vi "4-20mA Module (Main).vi"(7 "Name of Parent Panel":string="Main.vi", 9 "New Center Coords":T1={"Horizontal"=470, "Vertical"=200}, 10 "Config":variant, 11 "Main UI Message Queue":refnum<queue>) -> ()   [LabVIEW 2018, in "4-20mA Module.lvlib"]
doc: "This Continuous Measurement sample project is based on the Queued Message Handler template.\n\nThe Event Handling Loop generates messages based on user interface actions.\n\nThe Message Handling Loop processes messages generated by the Event Handling Loop, or by other messages. There are also Acquisition and Logging message handling loop subVIs, and a chart updating loop."
uses:
  4-20mA Module.lvlib
  support/Message Queue/Message Cluster.ctl
  <vilib>/Utility/miscctls.llb/LVPoint32TypeDef.ctl
  controls/UI Data.ctl
  controls/UI State.ctl
  Controls/4-20mA Module State Cluster.ctl
  Controls/4-20mA Module Config Cluster.ctl
  Controls/4-20mA Module Settings Cluster.ctl
  Pressure Transmitter/Pressure Transmitter Device Settings.ctl
  Pressure Reg Module/Pressure Regulator Device Settings.ctl
  Measure Instrument/State Enum.ctl
  Controls/4-20mA Display Cluster.ctl
  Tag VIs/Tag FGV Operation Enum.ctl
  Sequencing/Squence Update Cluster.ctl
  support/Message Queue/Enqueue Message (Single).vi
  <vilib>/Utility/error.llb/Error Cluster From Error Code.vi
  <vilib>/ErrorRing/Error Ring.xnode
  support/User Event - Stop/User Event - Stop.lvlib
  support/Support Library.lvlib
  support/Message Queue/Message Queue.lvlib
  Measure Instrument/4-20mA Module Engine.lvlib
  Sequencing/Sequencing Library.lvlib
  Pressure Transmitter/Pressure Transmitter Library.lvlib
  Pressure Reg Module/Pressure Regulator Library.lvlib
  Shared Variables/Dynamic Shared Variables.lvlib
  Measure Instrument/Feed Module Engine.lvlib
  support/Command Log VIs/Command Logging.lvlib
panel:
  in  "Settings Dialog Button":bool
  out "Image Status":u16(ring)=2
  out "Input Channel":string
  out "Output":dbl caption="mA" format="%.2f"
  out "Input":dbl caption="mA" format="%.2f"
  out "Log File path":path
  out "Status":string
  in  "Exit":bool
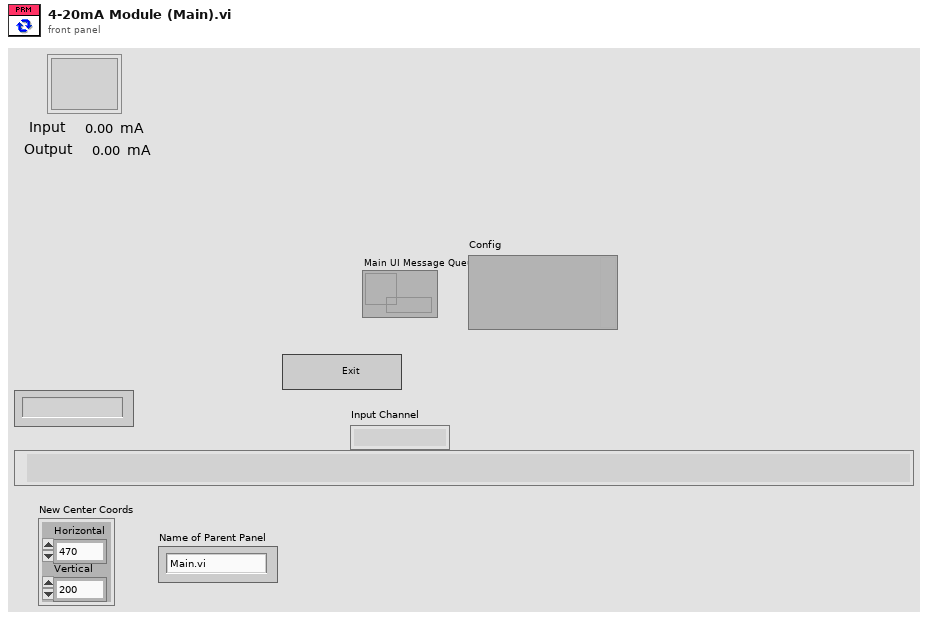
[diagram p1: front panel]
types:
  T1 = typedef "LVPoint32TypeDef.ctl" = cluster{"Horizontal":i32, "Vertical":i32}
  T2 = typedef "4-20mA Module.lvlib/4-20mA Module Config Cluster.ctl" = cluster{"GUID":string, "Drop Coords":T1, "Process Name":string, "Settings":T3, "Settings Load Count":i32}
  T3 = typedef "4-20mA Module.lvlib/4-20mA Module Settings Cluster.ctl" = cluster{"Cycle Period":dbl, "PID 2 Parameters":cluster{"Input Device":enum16{"Default", "4-20mA"}, "Output Device":enum16{"Default", "Equilibar Pressure Reg", "Flow Regulator"}, "Setpoint":dbl, "PID gains":cluster{"proportional gain (Kc)":dbl, "integral time (Ti, min)":dbl, "derivative time (Td, min)":dbl}, "output range":cluster{"output low":dbl, "output high":dbl}}, "Manual Entry":dbl, "Auto?":bool, "4-20mA Input Settings":T4, "4-20mA Out Settings":T5, "Input Channel Tag Name ":string}
  T4 = typedef "Pressure Transmitter Library.lvlib/Pressure Transmitter Device Settings.ctl" = cluster{"Input Channel ":u16}
  T5 = typedef "Pressure Regulator Library.lvlib/Pressure Regulator Device Settings.ctl" = cluster{"Output DAQ Task":refnum<k21>}
  T6 = typedef "4-20mA Module.lvlib/4-20mA Module State Cluster.ctl" = cluster{"PRM Config":T2, "State":T7, "Start Time":timestamp, "Current Time":timestamp, "First Iteration":bool, "Data":cluster{"4-20mA Input":dbl, "PID 2 Process Variable":dbl, "PID 2 Output":dbl, "4-20mA Output":dbl}}
  T7 = typedef "Feed Module.lvlib/Feed Module Engine.lvlib/State Enum.ctl" = enum16{"Measuring", "Idle", "Paused"}
  T8 = typedef "UI State.ctl" = enum16{"Idle", "Acquiring and Logging", "Waiting for Exit", "Waiting for Exit (Acq Stopped)", "Waiting for Exit (Log Stopped)", "Waiting for Stop", "Waiting for Stop (Acq Stopped)", "Waiting for Stop (Log Stopped)"}
  T9 = typedef "UI Data.ctl" = cluster{"Start Ref":refnum<vi>, "Trigger Ref":refnum<vi>, "Stop Ref":refnum<vi>, "Settings Ref":refnum<vi>, "Status Ref":refnum<vi>, "Exit Ref":refnum<vi>, "Data Ref":refnum<vi>}
  T10 = typedef "4-20mA Module.lvlib/4-20mA Message Queues.ctl" = cluster{"UI":refnum<queue>, "Engine":refnum<queue>, "PR Display":refnum<queue>, "Setting Display":refnum<queue>}
  T11 = typedef "4-20mA Module.lvlib/4-20mA Display Cluster.ctl" = cluster{"Input 4-20":dbl, "Output 4-20":dbl, "Cycle Period":dbl, "Status":enum16{"Off", "On", "Not Initialized"}}
  T12 = typedef "Tag FGV Operation Enum.ctl" = enum16{"Init", "Set Notification Queue", "Create Tag", "Commit", "Write Tag (Numeric)", "Write Tag (Boolean)", "Read All Tags", "Read One Tag", "Delete Tag Category", "Set Alarm Parameters (Numeric)", "Set Alarm Parameters (Boolean)", "Enable All Alarms", "Disable All Alarms", "Delete All Tags", "Read Alarms", "Ack Alarm"}
  T13 = cluster{"Shift":bool, "Ctrl":bool, "Alt":bool, "Cmd":bool, "Opt":bool}
  T14 = typedef "Sequencing Library.lvlib/Squence Update Cluster.ctl" = cluster{"Auto?":bool, "Manual Entry":dbl, "Setpoint":dbl}
  T15 = enum8{"Enabled", "Disabled", "Disabled and Grayed Out"}
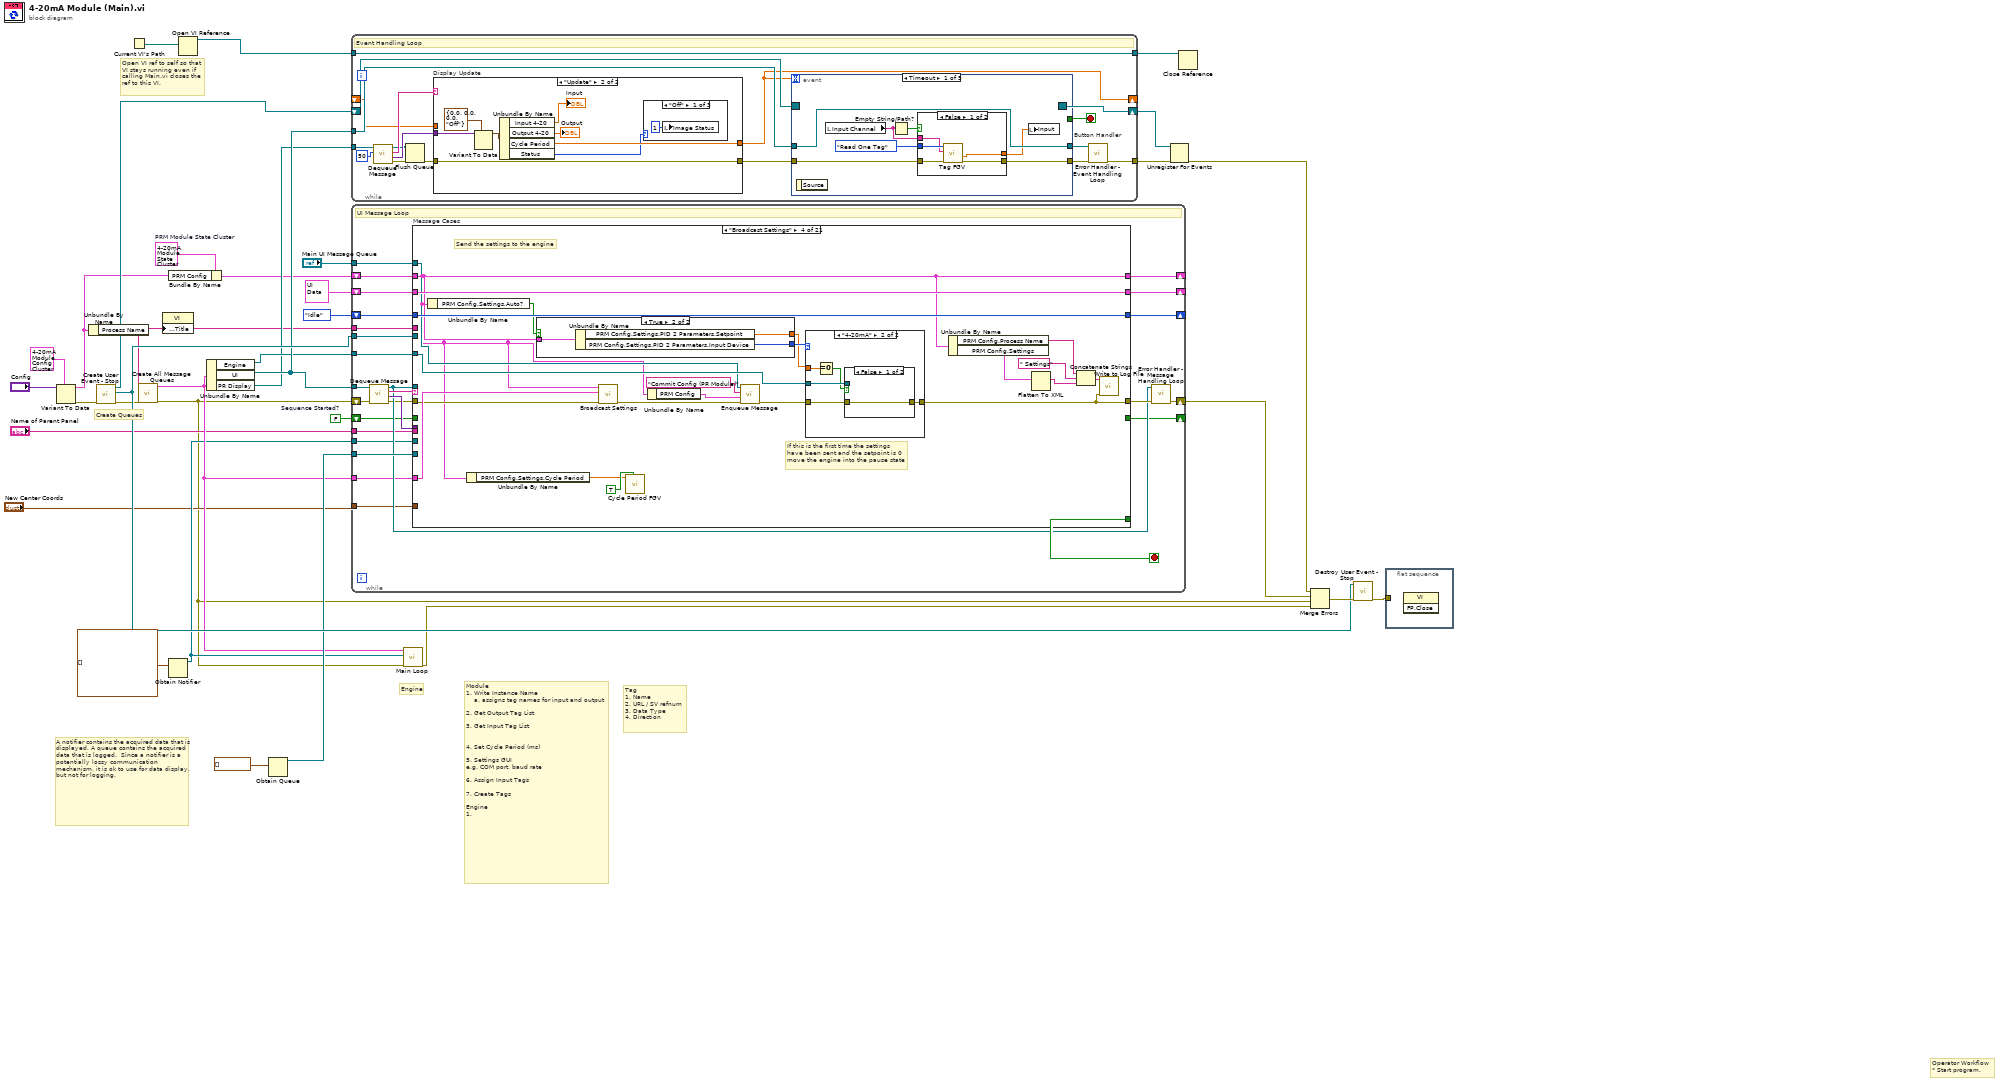
[diagram p0: block diagram]
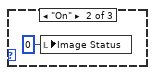
[diagram p3: hidden frame]
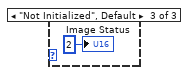
[diagram p4: hidden frame]
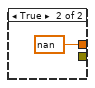
[diagram p5: hidden frame]
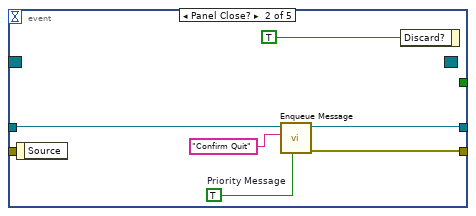
[diagram p6: hidden frame]
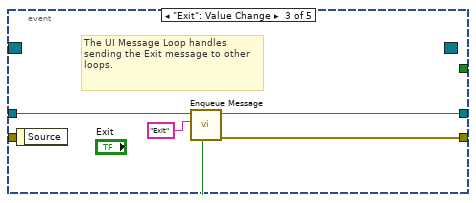
[diagram p7: hidden frame]
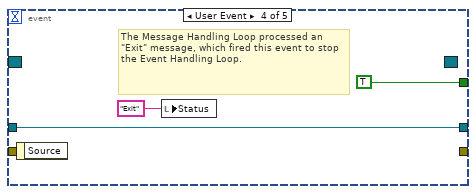
[diagram p8: hidden frame]
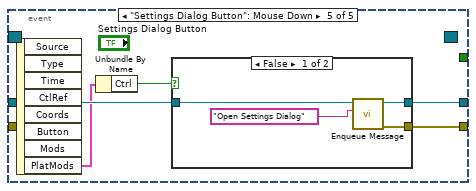
[diagram p9: hidden frame]
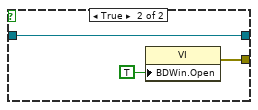
[diagram p10: hidden frame]
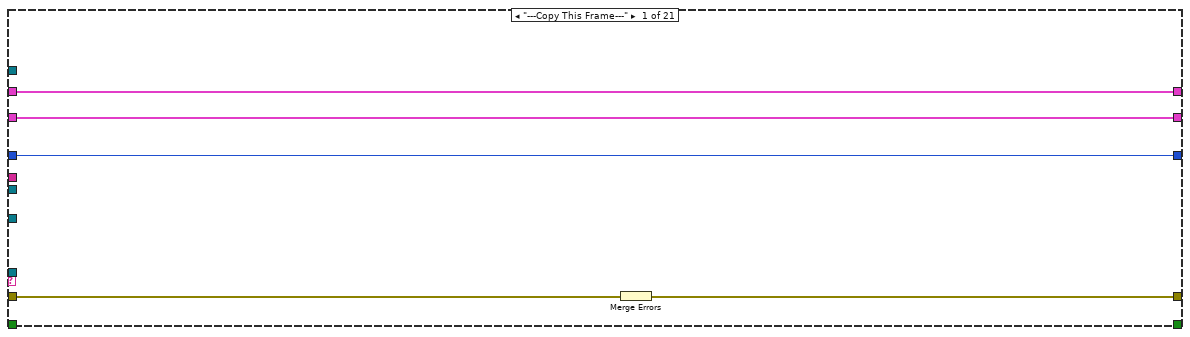
[diagram p11: hidden frame]
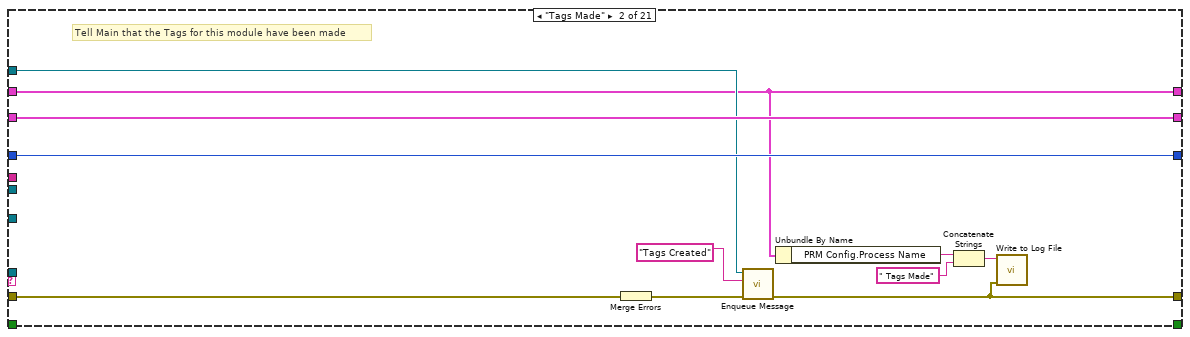
[diagram p12: hidden frame]
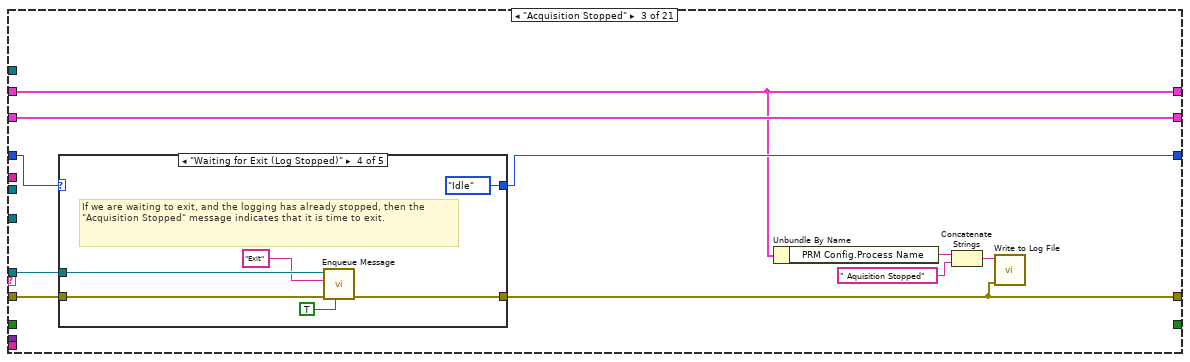
[diagram p13: hidden frame]
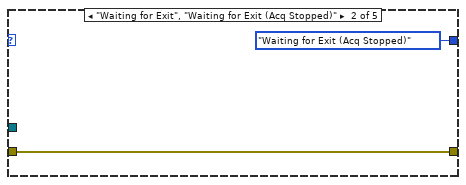
[diagram p15: hidden frame]
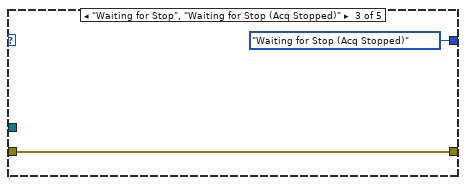
[diagram p16: hidden frame]
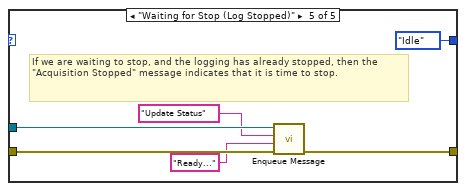
[diagram p17: hidden frame]
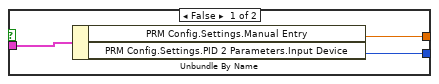
[diagram p18: hidden frame]
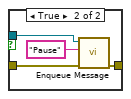
[diagram p20: hidden frame]
diagram:
  w5 = FALSE  # Sequence Started?
  w11 = T6 {"PRM Config"={"GUID"="", "Drop Coords"={"Horizontal"=0, "Vertical"=0}, "Process Name"="", "Settings"={"Cycle Period"=500.0, "PID 2 Parameters"={"Input Device"=enum."Default", "Output Device"=enum."Default", "Setpoint"=0.0, "PID gains"={"proportional gain (Kc)"=1.0, "integral time (Ti, min)"=0.01, "derivative time (Td, min)"=0.0}, "output range"={"output low"=0.0, "output high"=100.0}}, "Manual Entry"=0.0, "Auto?"=TRUE, "4-20mA Input Settings"={"Input Channel "=0}, "4-20mA Out Settings"={"Output DAQ Task"=""}, "Input Channel Tag Name "=""}, "Settings Load Count"=0}, "State"=enum."Idle", "Start Time"=timestamp(0 s since 1904-01-01), "Current Time"=timestamp(0 s since 1904-01-01), "First Iteration"=FALSE, "Data"={"4-20mA Input"=0.0, "PID 2 Process Variable"=0.0, "PID 2 Output"=0.0, "4-20mA Output"=0.0}}  # PRM Module State Cluster
  # "Create Queues"
  # "Open VI ref to self so that\nVI stays running even if\ncalling Main.vi closes the\nref to this VI."
  # "Engine"
  # "Operator Workflow\n* Start program."
  # "Module \n1. Write Instance Name\n    a. assigns tag names for input and output\n\n2. Get Output Tag List\n\n3. Get Input Tag List\n\n\n4. Set Cycle Period (ms)\n\n5. Settings GUI\ne.g. COM port, baud rate\n\n6. Assign Input Tags\n\n7. Create Tags\n\nEngine\n1."
  # "Tag\n1. Name\n2. URL / SV refnum\n3. Data Type\n4. Direction"
  # "A notifier contains the acquired data that is displayed. A queue contains the acquired data that is logged.  Since a notifier is a potentially lossy communication mechanism, it is ok to use for data display, but not for logging."
  n1 = Variant To Data(type=T2 {"GUID"="", "Drop Coords"={"Horizontal"=0, "Vertical"=0}, "Process Name"="", "Settings"={"Cycle Period"=500.0, "PID 2 Parameters"={"Input Device"=enum."Default", "Output Device"=enum."Default", "Setpoint"=0.0, "PID gains"={"proportional gain (Kc)"=1.0, "integral time (Ti, min)"=0.01, "derivative time (Td, min)"=0.0}, "output range"={"output low"=0.0, "output high"=100.0}}, "Manual Entry"=0.0, "Auto?"=TRUE, "4-20mA Input Settings"={"Input Channel "=0}, "4-20mA Out Settings"={"Output DAQ Task"=""}, "Input Channel Tag Name "=""}, "Settings Load Count"=0} ("Feed Module Config"), Variant="Config") -> (data=w13:T2, error out=w14:errorcluster)  [unwired: 1 in]
  n2 = Unbundle By Name(w13) -> ("Process Name"=w8:string)
  n3 = call "Create User Event - Stop.vi"("error in (no error)"=w14) -> ("error out"=w30:errorcluster, "User Event - Stop"=w31:refnum<user-event>, "Stop Event Registration Refnum"=w32:refnum<event-registration>)  [unwired: 8 in]
  n4 = Current VI's Path() -> (path=w15:path)
  n5 = call "Create All Message Queues.vi"("error in (no error)"=w30, "Process Name"=w8) -> ("error out"=w4:errorcluster, "Message Queues"=w19:T10)  [unwired: 8 in]
  n6 = property class="VI"("Front Panel.Title"=w8) -> ()  [unwired: 2 in, 2 out]
  n7 = Bundle By Name(cluster=w11, "PRM Config"=w13) -> (w1:T6)
  n8 = Obtain Notifier(notification data type=waveform(dbl)[] []) -> (notifier out=w18:refnum<notifier>)  [unwired: 3 in, 2 out]
  n9 = Open VI Reference(vi path=w15) -> (vi reference=w16:refnum<vi>)  [unwired: 5 in, 1 out]
  n10 = Unbundle By Name(w19) -> ("Engine"=w22:refnum<queue>, "UI"=w26:refnum<queue>, "PR Display"=w10:refnum<queue>)
  n11 = Obtain Queue(element data type=waveform(dbl)[] []) -> (queue out=w21:refnum<queue>)  [unwired: 4 in, 2 out]
  n12 = while {
    tunnel: w26 -> [w47]
    tunnel: [w49] -> w34
    shift-right: [w48] -> w28
    shift-left: w32 -> [w53]
    tunnel: [w46] -> w17
    tunnel: w16 -> [w46]
    tunnel: w10 -> [w45]
    shift-right: [w42] -> _
    shift-left: _ -> [w41]
    stop <- w52 stop-if-true
    # "Event Handling Loop"
    n13 = call "Dequeue Message.vi"("timeout in ms (-1)"=50, "Message Queue"=w45) -> ("error out"=w38:errorcluster, "Message Data"=w43:variant, "Message"=w44:string, "dup Message Queue"=w39:refnum<queue>)  [unwired: 6 in]
    n14 = Flush Queue(queue=w39, error in (no error)=w38) -> (error out=w36:errorcluster)  [unwired: 2 out]
    n15 = case "Display Update" shown="\"Update\"" w44 {
      tunnel: w43 -> [_ w63]
      tunnel: [w55 w59] -> w42
      tunnel: w41 -> [w55 _]
      tunnel: [w54 w57] -> w37
      tunnel: w36 -> [w54 w57]
      frame "False", Default {
      }
      frame "Update" {
        n16 = Variant To Data(type=T11 {"Input 4-20"=0.0, "Output 4-20"=0.0, "Cycle Period"=0.0, "Status"=enum."Off"} ("PRM Display Cluster"), Variant=w63) -> (data=w62:T11)  [unwired: 1 in, 1 out]
        n17 = Unbundle By Name(w62) -> ("Input 4-20"=→"Input":dbl, "Output 4-20"=→"Output":dbl, "Cycle Period"=w59:dbl, "Status"=w56:enum16{"Off", "On", "Not Initialized"})
        n18 = case shown="\"Off\"" w56 {
          frame "Off" {
            n19 = local write "Image Status"(u16 1 ("Ring")) -> ()
          }
          frame "On" {
            n20 = local write "Image Status"(u16 0 ("Ring")) -> ()
          }
          frame "Not Initialized", Default {
            "Image Status" <- u16 2 ("Ring")
          }
        }
      }
    }
    n21 = event "Button Handler" shown="[0] Timeout" {
      selector: w53 -> [_ _ _ _ _]
      dyn-events: [_ _ _ _ _] -> w48
      timeout: w42 -> [_ _ _ _ _]
      tunnel: [_ _ _ TRUE ("Discard?") _] -> w52
      tunnel: w47 -> [w73 w82 w87 w91 w96]
      tunnel: [w67 w80 w90 _ w98] -> w50
      tunnel: [w73 w81 w86 w91 w97] -> w51
      tunnel: w37 -> [w68 _ _ _ _]
      event Timeout {
        n22 = event-data() -> ()  [unwired: 1 in, 1 out]
        n23 = local read "Input Channel"() -> (w69:string)
        n24 = Empty String/Path?(string/path=w69) -> (empty?=w72:bool)
        n25 = case shown="False" w72 {
          tunnel: Tag_FGV_Operation_Enum."Read One Tag" ("Operation") -> [w78 _]
          tunnel: [w77 nan ("Tag Value")] -> w70
          tunnel: [w76 _] -> w67
          tunnel: w69 -> [w75 _]
          tunnel: w68 -> [w74 _]
          frame False {
            n26 = call "Tag FGV.vi"("error in (no error)"=w74, "Tag Name"=w75, "Operation"=w78) -> ("error out"=w76:errorcluster, "Tag Value"=w77:dbl)  [unwired: 3 in, 4 out]
          }
          frame True {
          }
        }
        n27 = local write "Input"(w70) -> ()
      }
      event Panel Close? {
        w83 = TRUE  # Priority Message
        n28 = event-data() -> ()  [unwired: 1 in, 1 out]
        n29 = call-poly "Enqueue Message.vi"("Priority Message? (F)"=w83, "Message"="Confirm Quit", "Message Queue"=w82) -> ("error out"=w80:errorcluster, "dup Message Queue"=w81:refnum<queue>)  [unwired: 7 in]
        n30 = event-data("Discard?"=TRUE) -> ()  [unwired: 1 in, 1 out]
      }
      event "Exit": Value Change {
        w88 = TRUE  # Priority Message
        # "The UI Message Loop handles sending the Exit message to other loops."
        n31 = event-data() -> ()  [unwired: 1 in, 1 out]
        n32 = call-poly "Enqueue Message.vi"("Priority Message? (F)"=w88, "Message"="Exit", "Message Queue"=w87) -> ("error out"=w90:errorcluster, "dup Message Queue"=w86:refnum<queue>)  [unwired: 7 in]
      }
      event User Event {
        # "The Message Handling Loop processed an \"Exit\" message, which fired this event to stop the Event Handling Loop."
        n33 = event-data() -> ()  [unwired: 1 in, 1 out]
        n34 = local write "Status"("Exit" ("Exit String")) -> ()
      }
      event "Settings Dialog Button": Mouse Down {
        n35 = event-data() -> ("PlatMods"=w95:T13)  [unwired: 1 in, 7 out]
        n36 = Unbundle By Name(w95) -> ("Ctrl"=w94:bool)
        n37 = case shown="False" w94 {
          tunnel: [w102 w103] -> w98
          tunnel: [w101 w104] -> w97
          tunnel: w96 -> [w100 w104]
          frame False {
            n38 = call-poly "Enqueue Message.vi"("Message"="Open Settings Dialog", "Message Queue"=w100) -> ("error out"=w102:errorcluster, "dup Message Queue"=w101:refnum<queue>)  [unwired: 8 in]
          }
          frame True {
            n39 = property class="VI"("BDWin.Open"=TRUE ("Block Diagram Window:Open")) -> (error out=w103:errorcluster)  [unwired: 2 in, 1 out]
          }
        }
      }
    }
    n40 = call "Error Handler - Event Handling Loop.vi"("error in (no error)"=w50, "Message Queue"=w51) -> ("dup error in"=w49:errorcluster)  [unwired: 8 in, 1 out]
  }
  n41 = while {
    tunnel: w26 -> [w126]
    tunnel: w31 -> [w130]
    shift-right: [w121] -> w35
    shift-left: w4 -> [w129]
    shift-right: [w124] -> _
    shift-left: T9 {"Start Ref"=refnum, "Trigger Ref"=refnum, "Stop Ref"=refnum, "Settings Ref"=refnum, "Status Ref"=refnum, "Exit Ref"=refnum, "Data Ref"=refnum} ("Measurement UI Controls") -> [w125]
    tunnel: w18 -> [w111]
    tunnel: w21 -> [w123]
    shift-right: [w119] -> _
    shift-left: UI_State."Idle" ("UI State") -> [w113]
    tunnel: w22 -> [w118]
    tunnel: w19 -> [w110]
    tunnel: "Main UI Message Queue" -> [w114]
    tunnel: "Name of Parent Panel" -> [w117]
    tunnel: w8 -> [w116]
    tunnel: "New Center Coords" -> [w115]
    shift-right: [w108] -> _
    shift-left: w5 -> [w109]
    shift-right: [w106] -> _
    shift-left: w1 -> [w107]
    stop <- w131 stop-if-true
    # "UI Message Loop"
    n42 = call "Dequeue Message.vi"("error in (no error)"=w129, "Message Queue"=w126) -> ("error out"=w112:errorcluster, "Message Data"=w127:variant, "Message"=w128:string, "dup Message Queue"=w120:refnum<queue>)  [unwired: 6 in]
    n43 = case "Message Cases" shown="\"Broadcast Settings\"" w128 {
      selector: w128 -> [_ _ _ _ _ _ _ _ _ _ _ _ _ _ _ _ _ _ _ _ w565]
      tunnel: w120 -> [_ _ w153 _ w222 _ w278 w294 w326 w350 _ w388 w409 w419 w452 w472 _ _ w542 _ _]
      tunnel: w112 -> [w136 w147 w154 w192 w221 w248 w263 w293 w329 w354 w373 w383 _ w420 w449 w470 w496 w510 w527 w556 _]
      tunnel: [w135 w138 w149 w179 w216 w249 w255 w282 w317 w332 w373 w375 w396 w415 w451 w463 w502 w516 w543 w557 w566] -> w122
      tunnel: [_ _ _ _ _ _ _ _ _ TRUE _ _ _ _ _ _ _ _ _ _ _] -> w131
      tunnel: w127 -> [_ _ _ _ _ w251 _ _ w328 w338 _ _ w407 _ _ _ _ _ _ w555 _]
      tunnel: w130 -> [_ _ _ _ _ _ _ _ _ w353 _ _ _ _ _ _ _ _ _ _ _]
      tunnel: w125 -> [w134 w146 w157 w197 w224 w253 w275 w291 w330 w351 w372 w384 w413 w423 w457 w486 w501 w515 w539 w552 w567]
      tunnel: [w134 w146 w157 w197 w224 w253 w275 w291 w330 w351 w371 w384 w413 w423 w457 w486 w501 w515 w539 w552 w567] -> w124
      tunnel: w123 -> [_ _ _ _ _ _ _ _ _ w345 _ _ _ _ _ _ _ _ _ _ _]
      tunnel: w113 -> [w133 w145 w156 w196 w223 w247 w264 _ w321 _ _ _ w412 w422 w442 _ _ _ w528 w547 w564]
      tunnel: [w133 w145 w155 w196 w220 w247 w265 UI_State."Acquiring and Logging" ("UI State") w321 UI_State."Idle" ("UI State") UI_State."Idle" ("UI State") UI_State."Idle" ("UI State") w412 w421 w442 UI_State."Acquiring and Logging" ("UI State") UI_State."Acquiring and Logging" ("UI State") UI_State."Acquiring and Logging" ("UI State") w529 w547 w564] -> w119
      tunnel: w118 -> [_ _ _ w191 _ _ w262 _ _ w343 _ _ _ _ _ _ w499 w513 w526 _ _]
      tunnel: w117 -> [_ _ _ _ _ _ _ _ _ _ _ w382 _ _ _ _ _ _ _ _ _]
      tunnel: w116 -> [_ _ _ _ _ _ _ _ _ _ _ w379 _ _ _ _ _ _ _ _ _]
      tunnel: w115 -> [_ _ _ _ _ _ _ _ _ _ _ w381 _ _ _ _ _ _ _ _ _]
      tunnel: w114 -> [_ w143 _ w184 _ _ _ _ _ w336 _ _ _ _ _ _ _ _ _ _ _]
      tunnel: w111 -> [_ _ _ _ _ _ _ _ _ w349 _ _ _ _ _ _ _ _ _ _ _]
      tunnel: w110 -> [_ _ _ w195 _ _ _ _ _ _ _ _ _ _ w443 _ _ _ _ _ _]
      tunnel: w107 -> [w132 w137 w148 w178 w215 w246 w254 w281 w316 w331 w364 w374 w411 w414 w450 w464 w494 w508 w522 w546 w563]
      tunnel: w109 -> [_ _ _ _ _ _ _ w290 _ _ _ _ _ _ _ _ _ _ _ _ _]
      tunnel: [_ _ _ _ _ _ _ w287 _ _ _ _ _ _ _ _ _ _ _ _ _] -> w108
      tunnel: [w132 w137 w148 w178 w215 w246 w254 w281 w316 w331 w364 w374 w395 w414 w445 w464 w494 w508 w522 w546 w563] -> w106
      frame "---Copy This Frame---" {
        # "Duplicate this frame when creating new messages.  Change this comment in the duplicated frame to describe this message."
        n44 = Merge Errors(w136) -> (w135:errorcluster)
      }
      frame "Tags Made" {
        # "Tell Main that the Tags for this module have been made"
        # "Duplicate this frame when creating new messages.  Change this comment in the duplicated frame to describe this message."
        n45 = Merge Errors(w147) -> (w142:errorcluster)
        n46 = call-poly "Enqueue Message.vi"("error in (no error)"=w142, "Message"="Tags Created", "Message Queue"=w143) -> ("error out"=w138:errorcluster)  [unwired: 7 in, 1 out]
        n47 = Unbundle By Name(w137) -> ("PRM Config.Process Name"=w141:string)
        n48 = Concatenate Strings(w141, " Tags Made" ("text")) -> (w139:string)
        n49 = call "Write to Log File.vi"("error in"=w138, "text"=w139) -> ()  [unwired: 9 in, 1 out]
      }
      frame "Acquisition Stopped" {
        # "Logic for determining what action to take when the acquisition has stopped."
        n50 = case shown="\"Waiting for Exit (Log Stopped)\"" w156 {
          selector: w156 -> [w159 _ _ _ _]
          tunnel: [w159 UI_State."Waiting for Exit (Acq Stopped)" ("UI State") UI_State."Waiting for Stop (Acq Stopped)" ("UI State") UI_State."Idle" ("UI State") UI_State."Idle" ("UI State")] -> w155
          tunnel: w154 -> [w158 w160 w162 w168 w174]
          tunnel: [w158 w160 w162 w167 w173] -> w149
          tunnel: w153 -> [_ _ _ w166 w172]
          frame Default {
          }
          frame "Waiting for Exit", "Waiting for Exit (Acq Stopped)" {
          }
          frame "Waiting for Stop", "Waiting for Stop (Acq Stopped)" {
          }
          frame "Waiting for Exit (Log Stopped)" {
            # "If we are waiting to exit, and the logging has already stopped, then the \"Acquisition Stopped\" message indicates that it is time to exit."
            n51 = call-poly "Enqueue Message.vi"("Priority Message? (F)"=TRUE, "error in (no error)"=w168, "Message"="Exit", "Message Queue"=w166) -> ("error out"=w167:errorcluster)  [unwired: 6 in, 1 out]
          }
          frame "Waiting for Stop (Log Stopped)" {
            # "If we are waiting to stop, and the logging has already stopped, then the \"Acquisition Stopped\" message indicates that it is time to stop."
            n52 = call-poly "Enqueue Message.vi"("error in (no error)"=w174, "Message Data"="Ready..." ("Message"), "Message"="Update Status", "Message Queue"=w172) -> ("error out"=w173:errorcluster)  [unwired: 6 in, 1 out]
          }
        }
        n53 = Unbundle By Name(w148) -> ("PRM Config.Process Name"=w152:string)
        n54 = Concatenate Strings(w152, " Aquisition Stopped" ("text")) -> (w150:string)
        n55 = call "Write to Log File.vi"("error in"=w149, "text"=w150) -> ()  [unwired: 9 in, 1 out]
      }
      frame "Broadcast Settings" {
        # "If this is the first time the settings\nhave been sent and the setpoint is 0 \nmove the engine into the pause state"
        # "Send the settings to the engine"
        # "Send the 'Update Settings' message to the Logging and Acquisition message loops."
        n56 = Unbundle By Name(w178) -> ("PRM Config.Settings.Auto?"=w188:bool)
        n57 = Unbundle By Name(w178) -> ("PRM Config.Settings.Cycle Period"=w193:dbl)
        n58 = case shown="True" w188 {
          tunnel: [w198 w203] -> w190
          tunnel: [w199 w202] -> w189
          tunnel: w178 -> [w200 w201]
          frame False {
            n59 = Unbundle By Name(w200) -> ("PRM Config.Settings.Manual Entry"=w199:dbl, "PRM Config.Settings.PID 2 Parameters.Input Device"=w198:enum16{"Default", "4-20mA"})
          }
          frame True {
            n60 = Unbundle By Name(w201) -> ("PRM Config.Settings.PID 2 Parameters.Setpoint"=w202:dbl, "PRM Config.Settings.PID 2 Parameters.Input Device"=w203:enum16{"Default", "4-20mA"})
          }
        }
        n61 = call "Broadcast Settings.vi"("error in (no error)"=w192, "Message Queues"=w195, "PRM Module State Cluster"=w178) -> ("error out"=w186:errorcluster)  [unwired: 8 in]
        n62 = call "Cycle Period FGV.vi"("Write"=TRUE, "Cycle Period In (ms)"=w193) -> ()  [unwired: 8 in, 2 out]
        n63 = Unbundle By Name(w178) -> ("PRM Config"=w183:T2)
        n64 = call-poly "Enqueue Message.vi"("error in (no error)"=w186, "Message Data"=w183, "Message"="Commit Config (PR Module)", "Message Queue"=w184) -> ("error out"=w185:errorcluster)  [unwired: 6 in, 1 out]
        n65 = case shown="\"4-20mA\"" w190 {
          tunnel: w185 -> [w204 w209]
          tunnel: w191 -> [_ w208]
          tunnel: [w204 w207] -> w179
          tunnel: w189 -> [_ w206]
          frame "Default", Default {
          }
          frame "4-20mA" {
            n66 = Equal To 0?(x=w206) -> (x = 0?=w205:bool)
            n67 = case shown="False" w205 {
              tunnel: w209 -> [w210 w214]
              tunnel: w208 -> [_ w213]
              tunnel: [w210 w212] -> w207
              frame False {
              }
              frame True {
                n68 = call-poly "Enqueue Message.vi"("error in (no error)"=w214, "Message"="Pause", "Message Queue"=w213) -> ("error out"=w212:errorcluster)  [unwired: 7 in, 1 out]
              }
            }
          }
        }
        n69 = Unbundle By Name(w178) -> ("PRM Config.Process Name"=w182:string, "PRM Config.Settings"=w177:T3)
        n70 = Flatten To XML(anything=w177) -> (xml string=w176:string)
        n71 = Concatenate Strings(w182, " Settings" ("text"), w176) -> (w180:string)
        n72 = call "Write to Log File.vi"("error in"=w179, "text"=w180) -> ()  [unwired: 9 in, 1 out]
      }
      frame "Confirm Quit" {
        # "Confirm Quit - Message that can confirm whether or not the user wants to exit the application."
        n73 = case shown="\"Acquiring and Logging\"" w223 {
          tunnel: w222 -> [w229 w235]
          tunnel: w221 -> [w228 w233]
          tunnel: [w225 w232] -> w216
          tunnel: [UI_State."Idle" ("UI State") w231] -> w220
          frame Default {
            # "If 'Confirm Quit' comes in while the system is idle, there is no need for a confirmation message."
            n74 = call-poly "Enqueue Message.vi"("Priority Message? (F)"=TRUE, "error in (no error)"=w228, "Message"="Exit", "Message Queue"=w229) -> ("error out"=w225:errorcluster)  [unwired: 6 in, 1 out]
          }
          frame "Acquiring and Logging" {
            n75 = Two Button Dialog(message="Are you sure you want to quit while the acquisition is running?" ("Confirm Quit Message"), 1:"No" ("No"), 2:"Yes" ("Yes")) -> (T button?=w234:bool)
            n76 = case shown="True" w234 {
              tunnel: w235 -> [_ w245]
              tunnel: w233 -> [w239 w244]
              tunnel: [w239 w243] -> w232
              tunnel: [UI_State."Acquiring and Logging" ("UI State") UI_State."Waiting for Exit" ("UI State")] -> w231
              frame False {
                # "User did not want to quit."
              }
              frame True {
                n77 = call-poly "Enqueue Message.vi"("error in (no error)"=w244, "Message"="Stop", "Message Queue"=w245) -> ("error out"=w243:errorcluster)  [unwired: 7 in, 1 out]
              }
            }
          }
        }
        n78 = Unbundle By Name(w215) -> ("PRM Config.Process Name"=w219:string)
        n79 = Concatenate Strings(w219, " Confirm Quit" ("text")) -> (w217:string)
        n80 = call "Write to Log File.vi"("error in"=w216, "text"=w217) -> ()  [unwired: 9 in, 1 out]
      }
      frame "Display Log File Path" {
        n81 = Variant To Data(error in=w248, type=path "", Variant=w251) -> (data=→"Log File path":path, error out=w249:errorcluster)
      }
      frame "E-Stop" {
        # "E-Stop pauses the engine"
        # "Message Acquisition and Logging loops to stop"
        # "Enable: Start, Exit, Settings\nDisable: Stop"
        # "Stop the pumps."
        n82 = Unbundle By Name(w275) -> ("Trigger Ref"=w266:refnum<vi>, "Stop Ref"=w267:refnum<vi>, "Start Ref"=w270:refnum<vi>, "Exit Ref"=w269:refnum<vi>, "Settings Ref"=w268:refnum<vi>)
        n83 = call-poly "Enqueue Message.vi"("error in (no error)"=w263, "Message Data"="Ready..." ("Ready..."), "Message"="Update Status", "Message Queue"=w278) -> ("error out"=w260:errorcluster)  [unwired: 6 in, 1 out]
        n84 = Build Array(w270, w269, w268) -> (w273:refnum<vi>[])
        n85 = Build Array(w266, w267) -> (w272:refnum<vi>[])
        n86 = call-poly "Enqueue Message.vi"("error in (no error)"=w260, "Message"="Pause", "Message Queue"=w262) -> ("error out"=w259:errorcluster)  [unwired: 7 in, 1 out]
        n87 = call "Set Enable State on Multiple Controls.vi"("Enable?"=FALSE, "Controls"=w272) -> ()  [unwired: 10 in]
        n88 = call "Set Enable State on Multiple Controls.vi"("Enable?"=TRUE, "Controls"=w273) -> ()  [unwired: 10 in]
        n89 = case shown="\"Waiting for Exit\"" w264 {
          selector: w264 -> [_ w280]
          tunnel: [UI_State."Waiting for Stop" ("UI State") w280] -> w265
          frame Default {
          }
          frame "Waiting for Exit" {
          }
        }
        n90 = Merge Errors(w259) -> (w255:errorcluster)
        n91 = Unbundle By Name(w254) -> ("PRM Config.Process Name"=w258:string)
        n92 = Concatenate Strings(w258, " E-STOP" ("text")) -> (w256:string)
        n93 = call "Write to Log File.vi"("error in"=w255, "text"=w256) -> ()  [unwired: 9 in, 1 out]
      }
      frame "Sequence Start" {
        # "Clear chart"
        # "Message Acquisition and Logging loops to start"
        # "Enable: Stop\nDisable: Start, Exit, Settings"
        # "Stop the pumps."
        n94 = Unbundle By Name(w291) -> ("Trigger Ref"=w298:refnum<vi>, "Stop Ref"=w299:refnum<vi>, "Start Ref"=w302:refnum<vi>, "Exit Ref"=w301:refnum<vi>, "Settings Ref"=w300:refnum<vi>, "Data Ref"=w296:refnum<vi>)
        n95 = property class="WFChart (strict)"(reference=w296, "History Data"=waveform(dbl)[][] []) -> ()  [unwired: 1 in, 2 out]
        n96 = Build Array(w302, w301, w300) -> (w305:refnum<vi>[])
        n97 = Build Array(w298, w299) -> (w304:refnum<vi>[])
        n98 = call-poly "Enqueue Message.vi"("error in (no error)"=w293, "Message"="Broadcast settings", "Message Queue"=w294) -> ("error out"=w288:errorcluster, "dup Message Queue"=w289:refnum<queue>)  [unwired: 7 in]
        n99 = call "Set Enable State on Multiple Controls.vi"("Enable?"=TRUE, "Controls"=w304) -> ()  [unwired: 10 in]
        n100 = call "Set Enable State on Multiple Controls.vi"("Enable?"=FALSE, "Controls"=w305) -> ()  [unwired: 10 in]
        n101 = case shown="False" w290 {
          selector: w290 -> [_ w312]
          tunnel: [w311 w312] -> w287
          tunnel: w288 -> [w310 w313]
          tunnel: w289 -> [w308 _]
          tunnel: [w307 w313] -> w286
          frame False {
            w311 = TRUE  # Sequence Started?
            n102 = call-poly "Enqueue Message.vi"("error in (no error)"=w310, "Message"="Start Loops", "Message Queue"=w308) -> ("error out"=w307:errorcluster)  [unwired: 7 in, 1 out]
          }
          frame True {
          }
        }
        n103 = Merge Errors(w286) -> (w282:errorcluster)
        n104 = Unbundle By Name(w281) -> ("PRM Config.Process Name"=w285:string)
        n105 = Concatenate Strings(w285, " Sequence Start" ("text")) -> (w283:string)
        n106 = call "Write to Log File.vi"("error in"=w282, "text"=w283) -> ()  [unwired: 9 in, 1 out]
      }
      frame "Error" {
        # "Stop if there is an error"
        # "Error - Check the error message data and respond accordingly. This message is sent by the \"Error Handler\" VIs at the end of each loop in this application."
        n107 = Variant To Data(error in=w329, type=errorcluster {"status"=FALSE, "code"=0, "source"=""} ("error out"), Variant=w328) -> (data=w314:errorcluster, error out=w323:errorcluster)
        n108 = call <vilib>:"Simple Error Handler.vi"("error in (no error)"=w314) -> ()  [unwired: 4 in, 5 out]
        n109 = call-poly "Enqueue Message.vi"("Priority Message? (F)"=TRUE, "Message"="Exit", "Message Queue"=w326) -> ("error out"=w322:errorcluster)  [unwired: 7 in, 1 out]
        n110 = Merge Errors(w322, w323) -> (w317:errorcluster)
        n111 = call <vilib>:"General Error Handler.vi"("error in (no error)"=w314) -> ("message"=w315:string)  [unwired: 10 in, 4 out]
        n112 = Unbundle By Name(w316) -> ("PRM Config.Process Name"=w320:string)
        n113 = Concatenate Strings(w320, " Error: " ("text"), w315) -> (w318:string)
        n114 = call "Write to Log File.vi"("error in"=w317, "text"=w318) -> ()  [unwired: 9 in, 1 out]
      }
      frame "Exit" {
        w340 = TRUE  # Delete Module?
        # "Don't check the error outs. The acquisition and logging queues may have already been released."
        # "Close references owned by the Main VI."
        # "Stop the VI"
        # "Exit - Fire the User Event to stop the Event Handling Loop.  Also send Exit messages to the Acquisition and Logging loops."
        n115 = Release Queue(queue=w350, error in (no error)=w354) -> (error out=w348:errorcluster)  [unwired: 1 in, 2 out]
        n116 = call "Fire User Event - Stop.vi"("User Event - Stop"=w353) -> ("error out"=w352:errorcluster)  [unwired: 10 in]
        n117 = Release Notifier(notifier=w349, error in (no error)=w348) -> (error out=w347:errorcluster)  [unwired: 1 in, 2 out]
        n118 = Variant To Data(type=w340, Variant=w338) -> (data=w339:bool, error out=w341:errorcluster)  [unwired: 1 in]
        n119 = Build Array(w343) -> (w342:refnum<queue>[])
        n120 = Release Queue(queue=w345, error in (no error)=w347) -> (error out=w346:errorcluster)  [unwired: 1 in, 2 out]
        n121 = Select(t=w340, s=w341, f=w339) -> (s? t:f=w337:bool)
        n122 = for {
          tunnel: w342 -> [w361] mode=indexing
          # "Send the engine the stop, exit"
          n123 = call-poly "Enqueue Message.vi"("Message"="Stop", "Message Queue"=w361) -> ("dup Message Queue"=w362:refnum<queue>)  [unwired: 8 in, 1 out]
          n124 = call-poly "Enqueue Message.vi"("Message"="Exit", "Message Queue"=w362) -> ()  [unwired: 8 in, 2 out]
        }
        n125 = case "Don't enqueue Delete Module if opening campaign because it\nwill already have been deleted and new config loaded and we create\na race condition." shown="True" w337 {
          tunnel: w331 -> [_ w358]
          tunnel: w336 -> [_ w356]
          frame False {
          }
          frame True {
            n126 = Unbundle By Name(w358) -> ("PRM Config.GUID"=w357:string)
            n127 = call-poly "Enqueue Message.vi"("Message Data"=w357, "Message"="Delete Module", "Message Queue"=w356) -> ()  [unwired: 7 in, 2 out]
          }
        }
        n128 = Merge Errors(w352, w346) -> (w332:errorcluster)
        n129 = Unbundle By Name(w331) -> ("PRM Config.Process Name"=w335:string)
        n130 = Concatenate Strings(w335, " Exit" ("text")) -> (w333:string)
        n131 = call "Write to Log File.vi"("error in"=w332, "text"=w333) -> ()  [unwired: 9 in, 1 out]
      }
      frame "Init UI Refs" {
        # "Enable: Start, Exit, Settings\nDisable: Stop"
        # "Init UI Refs - Store control references for UI controls.  Also enable/disable controls appropriately."
        n132 = property class="VI"("Front Panel.Closeable"=TRUE ("Front Panel Window:Closeable")) -> ()  [unwired: 2 in, 2 out]
        n133 = control-ref of="Status"() -> (w369:refnum<vi>)
        n134 = control-ref of="Exit"() -> (w366:refnum<vi>)
        n135 = Bundle By Name(cluster=w372, "Status Ref"=w369, "Exit Ref"=w366) -> (w371:T9)
        n136 = Build Array(w366) -> (w368:refnum<vi>[])
        n137 = call "Set Enable State on Multiple Controls.vi"("Enable?"=TRUE, "Controls"=w368) -> ()  [unwired: 10 in]
      }
      frame "Initialize" {
        # "Initialize - Get configuration settings, then message the UI to initialize, and broadcast the settings to the other message loops."
        n138 = property class="VI" props=["FP.State"]() -> (reference out=w380:refnum<vi>)  [unwired: 2 in, 2 out]
        n139 = call-poly "Enqueue Message.vi"("error in (no error)"=w383, "Message"="Init UI Refs", "Message Queue"=w388) -> ("error out"=w386:errorcluster, "dup Message Queue"=w387:refnum<queue>)  [unwired: 7 in]
        n140 = call-poly "Enqueue Message.vi"("error in (no error)"=w386, "Message"="Broadcast Settings", "Message Queue"=w387) -> ("error out"=w394:errorcluster, "dup Message Queue"=w393:refnum<queue>)  [unwired: 7 in]
        n141 = call "Make Child and Move.vi"("Process Name"=w379, "Name of Parent Panel"=w382, "New Center Coords"=w381, "VI in"=w380) -> ()  [unwired: 8 in]
        n142 = call-poly "Enqueue Message.vi"("error in (no error)"=w394, "Message Data"="Ready..." ("Ready..."), "Message"="Update Status", "Message Queue"=w393) -> ("error out"=w375:errorcluster)  [unwired: 6 in, 1 out]
        n143 = Unbundle By Name(w374) -> ("PRM Config.Process Name"=w378:string)
        n144 = Concatenate Strings(w378, " Initialize" ("text")) -> (w376:string)
        n145 = call "Write to Log File.vi"("error in"=w375, "text"=w376) -> ()  [unwired: 9 in, 1 out]
      }
      frame "Sequence Update" {
        # "Update the Sequence settings from the Sequence Dialog"
        # "Launch the Settings Dialog when the user clicks the 'Settings' button."
        n146 = Unbundle By Name(w411) -> ("PRM Config"=w410:T2)
        n147 = Variant To Data(type=T14 {"Auto?"=TRUE, "Manual Entry"=0.0, "Setpoint"=0.0} ("Cluster"), Variant=w407) -> (data=w406:T14)  [unwired: 1 in, 1 out]
        n148 = Unbundle By Name(w406) -> ("Auto?"=w405:bool, "Manual Entry"=w404:dbl, "Setpoint"=w403:dbl)
        n149 = Bundle By Name(cluster=w410, "Settings.Auto?"=w405, "Settings.Manual Entry"=w404, "Settings.PID 2 Parameters.Setpoint"=w403) -> (w400:T2)
        n150 = Bundle By Name(cluster=w411, "PRM Config"=w400) -> (w395:T6)
        n151 = call-poly "Enqueue Message.vi"("Message"="Broadcast Settings", "Message Queue"=w409) -> ("error out"=w402:errorcluster)  [unwired: 8 in, 1 out]
        n152 = Unbundle By Name(w395) -> ("PRM Config.Process Name"=w399:string)
        n153 = Merge Errors(w402) -> (w396:errorcluster)
        n154 = Concatenate Strings(w399, " Sequence Update" ("text")) -> (w397:string)
        n155 = call "Write to Log File.vi"("error in"=w396, "text"=w397) -> ()  [unwired: 9 in, 1 out]
      }
      frame "Logging Stopped" {
        # "Logic for determining what action to take when the logging has stopped."
        n156 = case shown="\"Waiting for Exit (Acq Stopped)\"" w422 {
          selector: w422 -> [w425 _ _ _ _]
          tunnel: [w425 UI_State."Waiting for Exit (Log Stopped)" ("UI State") UI_State."Waiting for Stop (Log Stopped)" ("UI State") UI_State."Idle" ("UI State") UI_State."Idle" ("UI State")] -> w421
          tunnel: w420 -> [w424 w426 w428 w434 w440]
          tunnel: [w424 w426 w428 w433 w439] -> w415
          tunnel: w419 -> [_ _ _ w432 w438]
          frame Default {
          }
          frame "Waiting for Exit", "Waiting for Exit (Log Stopped)" {
          }
          frame "Waiting for Stop", "Waiting for Stop (Log Stopped)" {
          }
          frame "Waiting for Exit (Acq Stopped)" {
            # "If we are waiting to exit, and the acquisition has already stopped, then the \"Logging Stopped\" message indicates that it is time to exit."
            n157 = call-poly "Enqueue Message.vi"("Priority Message? (F)"=TRUE, "error in (no error)"=w434, "Message"="Exit", "Message Queue"=w432) -> ("error out"=w433:errorcluster)  [unwired: 6 in, 1 out]
          }
          frame "Waiting for Stop (Acq Stopped)" {
            # "If we are waiting to stop, and the acquisition has already stopped, then the \"Logging Stopped\" message indicates that it is time to stop."
            n158 = call-poly "Enqueue Message.vi"("error in (no error)"=w440, "Message Data"="Ready..." ("Message"), "Message"="Update Status", "Message Queue"=w438) -> ("error out"=w439:errorcluster)  [unwired: 6 in, 1 out]
          }
        }
        n159 = Unbundle By Name(w414) -> ("PRM Config.Process Name"=w418:string)
        n160 = Concatenate Strings(w418, " Logging Stopped" ("text")) -> (w416:string)
        n161 = call "Write to Log File.vi"("error in"=w415, "text"=w416) -> ()  [unwired: 9 in, 1 out]
      }
      frame "Open Settings Dialog" {
        # "Keep track of how many times \nthe window has been opened"
        # "Duplicate this frame when creating new messages.  Change this comment in the duplicated frame to describe this message."
        n162 = Unbundle By Name(w450) -> ("PRM Config"=w454:T2)
        n163 = Unbundle By Name(w454) -> ("Settings Load Count"=w455:i32)
        n164 = Increment(x=w455) -> (x+1=w456:i32)
        n165 = Bundle By Name(cluster=w454, "Settings Load Count"=w456) -> (w453:T2)
        n166 = Bundle By Name(cluster=w450, "PRM Config"=w453) -> (w446:T6)
        n167 = call "Settings Dialog.vi"("error in (no error)"=w449, "UI State"=w442, "Message Queues"=w443, "PRM State Cluster In"=w446) -> ("error out"=w448:errorcluster, "Cancelled?"=w447:bool, "PRM State Cluster Out"=w445:T6)  [unwired: 4 in, 1 out]
        n168 = Unbundle By Name(w445) -> ("PRM Config.Settings.Input Channel Tag Name"=→"Input Channel":string)
        n169 = case shown="False" w447 {
          tunnel: w448 -> [w459 w462]
          tunnel: [w458 w462] -> w451
          tunnel: w452 -> [w461 _]
          frame False {
            n170 = call-poly "Enqueue Message.vi"("error in (no error)"=w459, "Message"="Broadcast Settings", "Message Queue"=w461) -> ("error out"=w458:errorcluster)  [unwired: 7 in, 1 out]
          }
          frame True {
          }
        }
      }
      frame "Start" {
        # "We only have one loop but i've kept this in anyway"
        # "Clear chart"
        # "Message Acquisition and Logging loops to start"
        # "Enable: Stop\nDisable: Start, Exit, Settings"
        # "Start - Enable/Disable buttons appropriately for an acquisition that has started, and update status display."
        n171 = Unbundle By Name(w486) -> ("Trigger Ref"=w477:refnum<vi>, "Stop Ref"=w478:refnum<vi>, "Start Ref"=w481:refnum<vi>, "Exit Ref"=w480:refnum<vi>, "Settings Ref"=w479:refnum<vi>, "Data Ref"=w469:refnum<vi>)
        n172 = disable-structure shown="Enabled" {
          disable-tunnel: [w490 w492] -> w473
          disable-tunnel: w472 -> [w489 w493]
          disable-tunnel: [w488 w493] -> w471
          disable-tunnel: w470 -> [w487 w492]
          frame Disabled {
            n173 = call-poly "Enqueue Message.vi"("error in (no error)"=w487, "Message"="Broadcast settings", "Message Queue"=w489) -> ("error out"=w490:errorcluster, "dup Message Queue"=w488:refnum<queue>)  [unwired: 7 in]
          }
          frame Enabled {
          }
        }
        n174 = property class="WFChart (strict)"(reference=w469, "History Data"=waveform(dbl)[][] []) -> ()  [unwired: 1 in, 2 out]
        n175 = Build Array(w481, w480, w479) -> (w484:refnum<vi>[])
        n176 = Build Array(w477, w478) -> (w483:refnum<vi>[])
        n177 = call "Set Enable State on Multiple Controls.vi"("Enable?"=TRUE, "Controls"=w483) -> ()  [unwired: 10 in]
        n178 = call "Set Enable State on Multiple Controls.vi"("Enable?"=FALSE, "Controls"=w484) -> ()  [unwired: 10 in]
        n179 = call-poly "Enqueue Message.vi"("error in (no error)"=w473, "Message"="Start Loops", "Message Queue"=w471) -> ("error out"=w474:errorcluster)  [unwired: 7 in, 1 out]
        n180 = Merge Errors(w474) -> (w463:errorcluster)
        n181 = Unbundle By Name(w464) -> ("PRM Config.Process Name"=w467:string)
        n182 = Concatenate Strings(w467, " Start" ("text")) -> (w465:string)
        n183 = call "Write to Log File.vi"("error in"=w463, "text"=w465) -> ()  [unwired: 9 in, 1 out]
      }
      frame "Start Loops" {
        # "I'm not entirly sure where we would have a second Process Name in a module but i'm leaving it for now"
        # "Message Acquisition and Logging loops to start"
        # "Start - Enable/Disable buttons appropriately for an acquisition that has started, and update status display."
        n184 = Build Array(w499) -> (w497:refnum<queue>[])
        n185 = Unbundle By Name(w494) -> ("PRM Config.Process Name"=w495:string)
        n186 = for {
          tunnel: w496 -> [w506]
          tunnel: [w505] -> w498 mode=indexing
          tunnel: w497 -> [w504] mode=indexing
          tunnel: w495 -> [w503]
          n187 = call-poly "Enqueue Message.vi"("error in (no error)"=w506, "Message Data"=w503, "Message"="Start", "Message Queue"=w504) -> ("error out"=w505:errorcluster)  [unwired: 6 in, 1 out]
        }
        n188 = property class="VI"("Front Panel.Title"=w495) -> ()  [unwired: 2 in, 2 out]
        n189 = Merge Errors(w498) -> (w502:errorcluster)
      }
      frame "Start Log" {
        # "I'm not entirly sure where we would have a second Process Name in a module but i'm leaving it for now"
        # "Message Acquisition and Logging loops to start"
        # "Start - Enable/Disable buttons appropriately for an acquisition that has started, and update status display."
        n190 = Build Array(w513) -> (w511:refnum<queue>[])
        n191 = Unbundle By Name(w508) -> ("PRM Config.Process Name"=w509:string)
        n192 = for {
          tunnel: w510 -> [w520]
          tunnel: [w519] -> w512 mode=indexing
          tunnel: w511 -> [w518] mode=indexing
          tunnel: w509 -> [w517]
          n193 = call-poly "Enqueue Message.vi"("error in (no error)"=w520, "Message Data"=w517, "Message"="Start Log", "Message Queue"=w518) -> ("error out"=w519:errorcluster)  [unwired: 6 in, 1 out]
        }
        n194 = property class="VI"("Front Panel.Title"=w509) -> ()  [unwired: 2 in, 2 out]
        n195 = Merge Errors(w512) -> (w516:errorcluster)
      }
      frame "Stop" {
        # "Stop Pauses the engine"
        # "Enable: Start, Exit, Settings\nDisable: Stop"
        # "Stop - Enable/Disable buttons appropriately for an acquisition that has stopped, and update status display."
        n196 = Unbundle By Name(w539) -> ("Trigger Ref"=w530:refnum<vi>, "Stop Ref"=w531:refnum<vi>, "Start Ref"=w534:refnum<vi>, "Exit Ref"=w533:refnum<vi>, "Settings Ref"=w532:refnum<vi>)
        n197 = call-poly "Enqueue Message.vi"("error in (no error)"=w527, "Message Data"="Ready..." ("Ready..."), "Message"="Update Status", "Message Queue"=w542) -> ("error out"=w525:errorcluster)  [unwired: 6 in, 1 out]
        n198 = Build Array(w534, w533, w532) -> (w537:refnum<vi>[])
        n199 = Build Array(w530, w531) -> (w536:refnum<vi>[])
        n200 = call-poly "Enqueue Message.vi"("error in (no error)"=w525, "Message"="Pause", "Message Queue"=w526) -> ("error out"=w523:errorcluster)  [unwired: 7 in, 1 out]
        n201 = call "Set Enable State on Multiple Controls.vi"("Enable?"=FALSE, "Controls"=w536) -> ()  [unwired: 10 in]
        n202 = call "Set Enable State on Multiple Controls.vi"("Enable?"=TRUE, "Controls"=w537) -> ()  [unwired: 10 in]
        n203 = case shown="\"Waiting for Exit\"" w528 {
          selector: w528 -> [_ w545]
          tunnel: [UI_State."Waiting for Stop" ("UI State") w545] -> w529
          frame Default {
          }
          frame "Waiting for Exit" {
          }
        }
        n204 = Merge Errors(w523) -> (w543:errorcluster)
      }
      frame "Update Status" {
        # "Update Display - Convert the message data to a string to display in the Status indicator."
        n205 = Unbundle By Name(w552) -> ("Trigger Ref"=w548:refnum<vi>, "Stop Ref"=w551:refnum<vi>)
        n206 = Variant To Data(error in=w556, type="", Variant=w555) -> (data=w549:string, error out=w553:errorcluster)
        "Status" <- w549
        n207 = property class="Bool"(reference=w551) -> ("DisabledEnum"=w550:T15)  [unwired: 1 in, 2 out]
        n208 = case shown="\"Enabled\"" w550 {
          tunnel: w549 -> [w560 _]
          tunnel: w548 -> [w561 _]
          frame "Enabled" {
            # "Disable the Force Trigger only while we are logging."
            n209 = Build Array(w561) -> (w562:refnum<vi>[])
            n210 = Not Equal?(x="Logging" ("Logging"), y=w560) -> (x != y?=w558:bool)
            n211 = call "Set Enable State on Multiple Controls.vi"("Enable?"=w558, "Controls"=w562) -> ()  [unwired: 10 in]
          }
          frame "Disabled", Default {
          }
        }
        n212 = Merge Errors(w553) -> (w557:errorcluster)
      }
      frame Default {
        # "'Default' case only runs if there is a message that isn't defined in any of the other cases.  Output a programming error."
        n213 = xnode "Error Ring"("parameter 0"=w565) -> ("error out"=w566:errorcluster)
      }
    }
    n214 = call "Error Handler - Message Handling Loop.vi"("error in (no error)"=w122, "Message Queue"=w120) -> ("dup error in"=w121:errorcluster)  [unwired: 8 in, 1 out]
  }
  n215 = call "Main Loop.vi"("error in (no error)"=w4, "Chart Notifier"=w18, "Message Queues"=w19) -> ("error out"=w20:errorcluster)  [unwired: 8 in]
  n216 = Unregister For Events(event registration refnum=w28, error in=w34) -> (error out=w29:errorcluster)
  n217 = Close Reference(reference=w17) -> ()  [unwired: 1 in, 1 out]
  n218 = Merge Errors(w29, w35, w4, w20) -> (w33:errorcluster)
  n219 = call "Destroy User Event - Stop.vi"("error in (no error)"=w33, "User Event - Stop"=w31) -> ("error out"=w6:errorcluster)  [unwired: 9 in]
  n220 = flat-sequence {
    tunnel: w6 -> [_]
    frame #0 {
      n221 = invoke class="VI" method="FP.Close"() -> ()  [unwired: 3 in, 3 out]
    }
  }
